vi "Update All Values.vi"(8 "error in (no error)":errorcluster, 10 "Values":refnum<class "Type.lvclass">[](array[class]), 11 "User in":refnum<class "User.lvclass">) -> (0 "error out":errorcluster, 3 "User out":refnum<class "User.lvclass">)   [LabVIEW 2020, in "Test.lvlib" / "User.lvclass"]
uses:
  User.lvclass
  <vilib>/IlluminatedG/IG Conditum/Conditum/Columns/String/String.lvclass
  <vilib>/IlluminatedG/IG Conditum/Conditum/Columns/Timestamp/Timestamp.lvclass
  <vilib>/IlluminatedG/IG Conditum/Conditum/Columns/Integer/Integer.lvclass
  <vilib>/IlluminatedG/IG Conditum/Conditum/Columns/Boolean/Boolean.lvclass
  <vilib>/IlluminatedG/IG Conditum/Conditum/Columns/Type/Type.lvclass
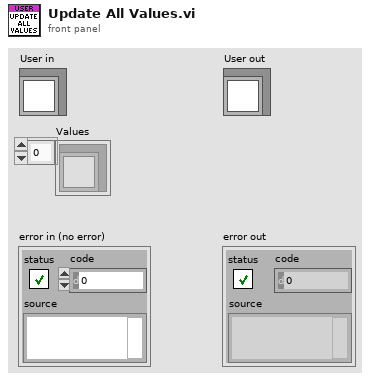
[diagram p1: front panel]
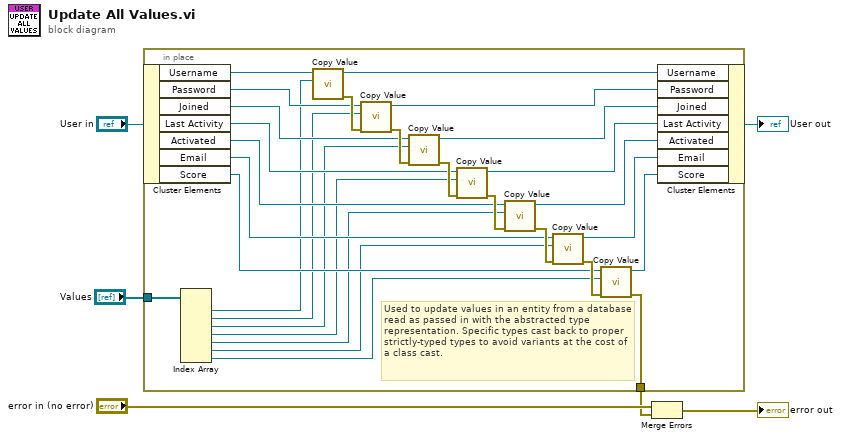
[diagram p0: block diagram]
diagram:
  n1 = in-place {
    in-place-border: "Values" -> [w33]
    in-place-border: [w7] -> w1
    # "Used to update values in an entity from a database read as passed in with the abstracted type representation. Specific types cast back to proper strictly-typed types to avoid variants at the cost of a class cast."
    n2 = in-place-cluster #1("User in") -> ("Username"=w35:refnum<class "String.lvclass">, "Password"=w26:refnum<class "String.lvclass">, "Joined"=w25:refnum<class "Timestamp.lvclass">, "Last Activity"=w24:refnum<class "Timestamp.lvclass">, "Activated"=w23:refnum<class "Boolean.lvclass">, "Email"=w22:refnum<class "String.lvclass">, "Score"=w21:refnum<class "Integer.lvclass">)
    n3 = Index Array(array=w33) -> (element #1=w14:refnum<class "Type.lvclass">, element #2=w13:refnum<class "Type.lvclass">, element #3=w12:refnum<class "Type.lvclass">, element #4=w11:refnum<class "Type.lvclass">, element #5=w10:refnum<class "Type.lvclass">, element #6=w9:refnum<class "Type.lvclass">, element #7=w8:refnum<class "Type.lvclass">)  [unwired: 7 in]
    n4 = call-dynamic "Copy Value.vi"("From"=w14, "String in"=w35) -> ("error out"=w30:errorcluster, "String out"=w34:refnum<class "String.lvclass">)  [unwired: 8 in]
    n5 = call-dynamic "Copy Value.vi"("error in (no error)"=w30, "From"=w13, "String in"=w26) -> ("error out"=w29:errorcluster, "String out"=w15:refnum<class "String.lvclass">)  [unwired: 7 in]
    n6 = call-dynamic "Copy Value.vi"("error in (no error)"=w29, "From"=w12, "Timestamp in"=w25) -> ("error out"=w28:errorcluster, "Timestamp out"=w16:refnum<class "Timestamp.lvclass">)  [unwired: 7 in]
    n7 = call-dynamic "Copy Value.vi"("error in (no error)"=w28, "From"=w11, "Timestamp in"=w24) -> ("error out"=w27:errorcluster, "Timestamp out"=w17:refnum<class "Timestamp.lvclass">)  [unwired: 7 in]
    n8 = call-dynamic "Copy Value.vi"("error in (no error)"=w27, "From"=w10, "Boolean in"=w23) -> ("error out"=w31:errorcluster, "Boolean out"=w18:refnum<class "Boolean.lvclass">)  [unwired: 7 in]
    n9 = call-dynamic "Copy Value.vi"("error in (no error)"=w31, "From"=w9, "String in"=w22) -> ("error out"=w32:errorcluster, "String out"=w19:refnum<class "String.lvclass">)  [unwired: 7 in]
    n10 = call-dynamic "Copy Value.vi"("error in (no error)"=w32, "From"=w8, "Integer in"=w21) -> ("error out"=w7:errorcluster, "Integer out"=w20:refnum<class "Integer.lvclass">)  [unwired: 7 in]
    n11 = in-place-cluster #1("Username"=w34, "Password"=w15, "Joined"=w16, "Last Activity"=w17, "Activated"=w18, "Email"=w19, "Score"=w20) -> (→"User out":refnum<class "User.lvclass">)
  }
  n12 = Merge Errors("error in (no error)", w1) -> (→"error out":errorcluster)
